vi "Stop Process.vi"(8 "error in (no error)":errorcluster, 11 "DAQ_Engine in":refnum<class "DAQ_Engine.lvclass">) -> (0 "error out":errorcluster, 3 "DAQ_Engine out":refnum<class "DAQ_Engine.lvclass">)   [LabVIEW 2019, in "DAQ_Engine.lvclass"]
doc: "Developed by Kevin Thompson\nkevin@thompsonengineering.net\n\nCopyright 2018\nThompson Engineering, LLC"
uses:
  DAQ_Engine.lvclass
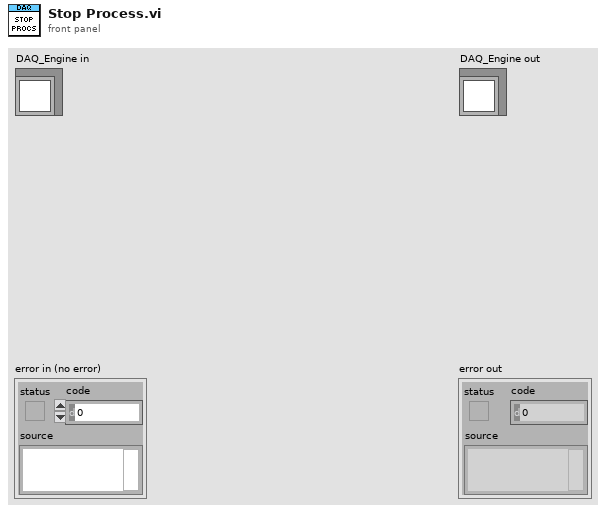
[diagram p1: front panel]
types:
  T1 = typedef "DAQ_Engine.lvclass/Public Events--cluster.ctl" = cluster{"DAQ_Engine.AsyncCmd Event":refnum<user-event>, "DAQ_Engine.AsyncMsg Event":refnum<user-event>, "stop process":refnum<user-event>, "DAQ_Engine.DAQStateChg Ev":refnum<user-event>, "DAQ_Engine.MeasSettingsChg Ev":refnum<user-event>, "DAQ_Engine.AcqModeChg Ev":refnum<user-event>}
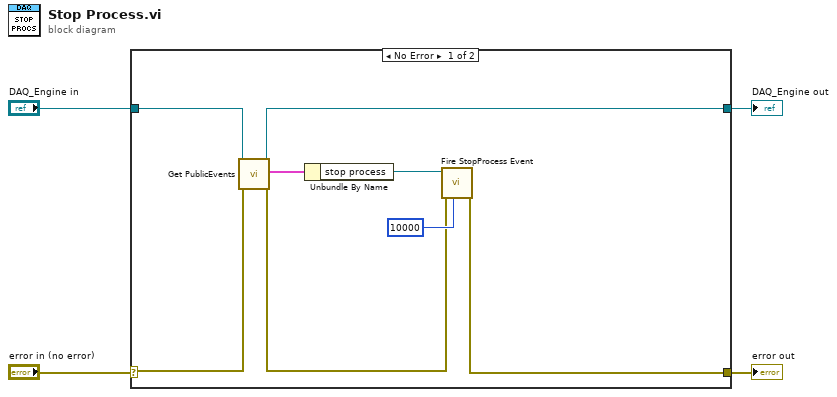
[diagram p0: block diagram]
diagram:
  n1 = case shown="No Error" "error in (no error)" {
    selector: "error in (no error)" -> [w6 w14]
    tunnel: [w12 w14] -> w3
    tunnel: [w8 w13] -> w1
    tunnel: "DAQ_Engine in" -> [w7 w13]
    frame No Error {
      n2 = call "Get PublicEvents.vi"("error in (no error)"=w6, "DAQ_Engine in"=w7) -> ("error out"=w5:errorcluster, "Public Events"=w10:T1, "DAQ_Engine out"=w8:refnum<class "DAQ_Engine.lvclass">)  [unwired: 7 in]
      n3 = Unbundle By Name(w10) -> ("stop process"=w9:refnum<user-event>)
      n4 = call "Fire StopProcess Event.vi"("timeout in ms (5000)"=10000, "error in (no error)"=w5, "Event in"=w9) -> ("error out"=w12:errorcluster)  [unwired: 5 in, 3 out]
    }
    frame Error {
    }
  }
  "error out" <- w3
  "DAQ_Engine out" <- w1
